vi "TRAJECTORY_CREATE_PATHFINDER_BEGIN.vi"() -> (0 "Path calculation error":errorcluster, 2 "Trajectory Items":i32, 3 "TotalTImeSecs":dbl)   [LabVIEW 2019]
uses:
  <vilib>/Rock Robotics/WPI/ThirdParty/JAS_Junk/JaciPathFinderLib/VIs/Waypoint.ctl
  <vilib>/Rock Robotics/WPI/ThirdParty/JAS_Junk/TrajLib/TRAJECTORY.ctl
  <vilib>/Rock Robotics/WPI/ThirdParty/JAS_Junk/TrajLib/TRAJ_STATE.ctl
  <vilib>/Rock Robotics/WPI/ThirdParty/JAS_Junk/TrajLib/POSE2D.ctl
  <vilib>/Rock Robotics/WPI/ThirdParty/JAS_Junk/TrajLib/TRANSLATION2D.ctl
  <vilib>/Rock Robotics/WPI/ThirdParty/JAS_Junk/TrajLib/ROTATION2D.ctl
  <vilib>/Rock Robotics/WPI/ThirdParty/JAS_Junk/TrajLib/Trajectory_Library.lvlib
  <vilib>/Rock Robotics/WPI/ThirdParty/JAS_Junk/JaciPathFinderLib/Pathfinder.lvlib
panel:
  out "TRAJECTORY":T1 {"TotalTImeSecs" format="%20.3f"}
  in  "Waypoints":T6[](array[typedef])=[{"x"=15.0, "y"=105.0, "angle"=-45.0}, {"x"=105.0, "y"=65.0, "angle"=0.0}, {"x"=210.0, "y"=106.0, "angle"=45.0}]
  in  "wheelbase_width":dbl=20.866
  in  "sample_count":i32=10000
  in  "Path Results\ndT":dbl=0.02 format="%7.3f"
  in  "max_jerk":dbl=50.0
  in  "max_acceleration":dbl=20.0
  in  "max_velocity":dbl=40.0
  # "TRAJECTORY CONFIGURATION"
  # "TRAJECTORY DEFINITION"
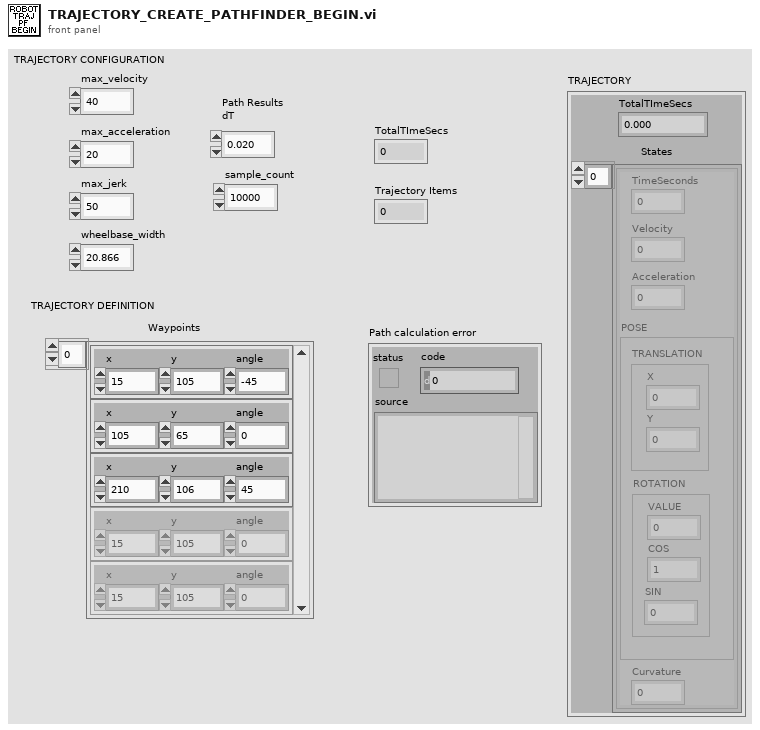
[diagram p1: front panel]
types:
  T1 = typedef "Trajectory_Library.lvlib/TRAJECTORY.ctl" = cluster{"TotalTImeSecs":dbl, "States":T2[]}
  T2 = typedef "Trajectory_Library.lvlib/TRAJ_STATE.ctl" = cluster{"TimeSeconds":dbl, "Velocity":dbl, "Acceleration":dbl, "POSE":T3, "Curvature":dbl}
  T3 = typedef "Trajectory_Library.lvlib/POSE2D.ctl" = cluster{"TRANSLATION":T4, "ROTATION":T5}
  T4 = typedef "Trajectory_Library.lvlib/TRANSLATION2D.ctl" = cluster{"X":dbl, "Y":dbl}
  T5 = typedef "Trajectory_Library.lvlib/ROTATION2D.ctl" = cluster{"VALUE":dbl, "COS":dbl, "SIN":dbl}
  T6 = typedef "Pathfinder.lvlib/Waypoint.ctl" = cluster{"x":dbl, "y":dbl, "angle":dbl}
  T7 = typedef "Pathfinder.lvlib/Segment.ctl" = cluster{"dt":dbl, "x":dbl, "y":dbl, "position":dbl, "velocity":dbl, "acceleration":dbl, "jerk":dbl, "heading":dbl}
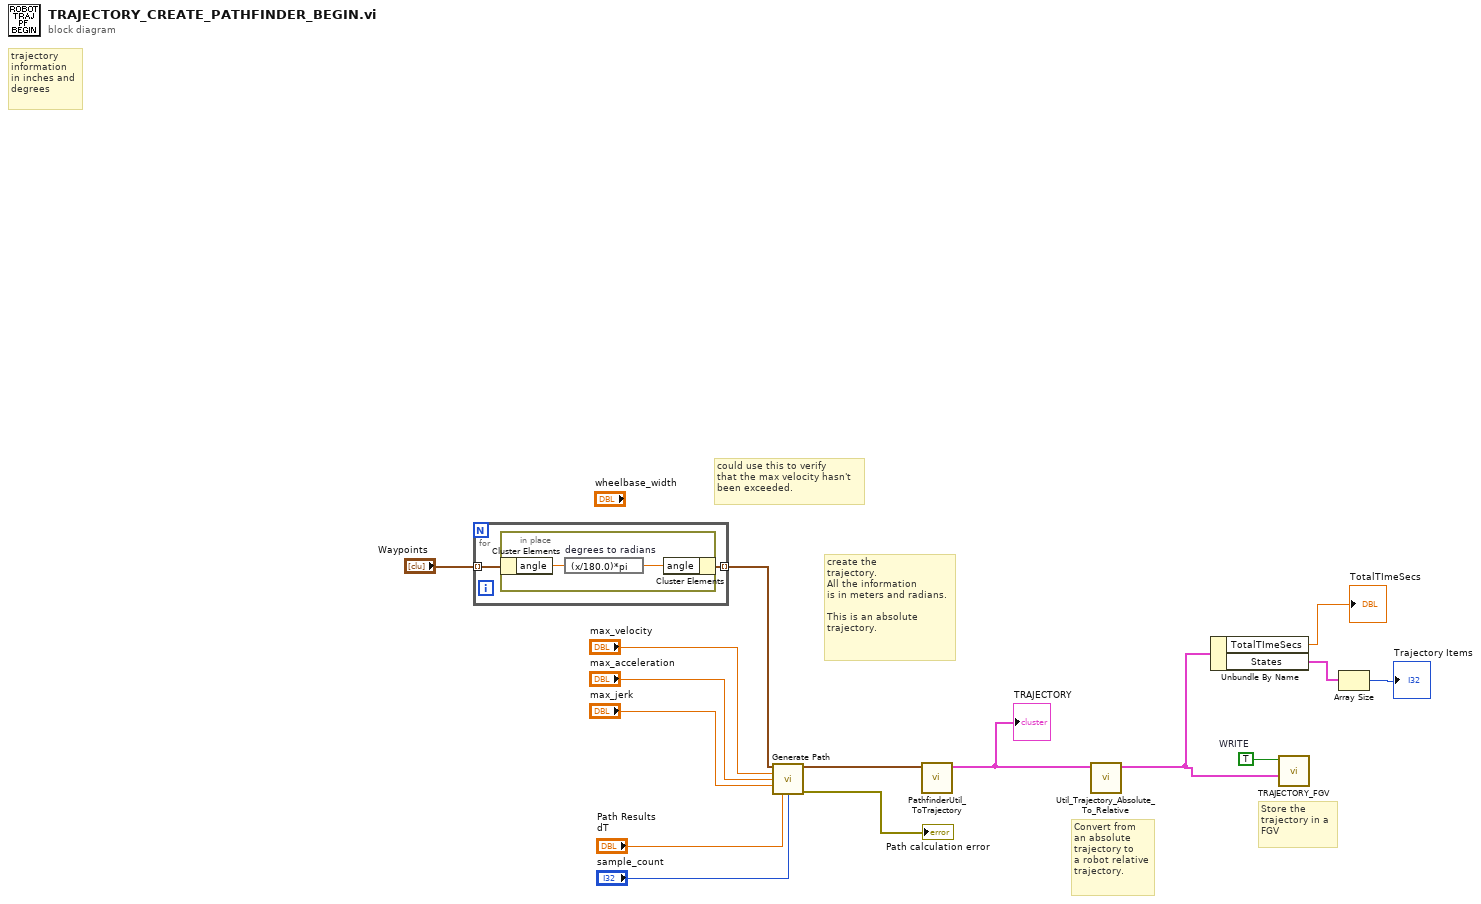
[diagram p0: block diagram]
diagram:
  w15 = TRUE  # WRITE
  # "could use this to verify\nthat the max velocity hasn't\nbeen exceeded."
  # "Store the\ntrajectory in a \nFGV"
  # "Convert from\nan absolute\ntrajectory to\na robot relative\ntrajectory."
  # "create the\ntrajectory.\nAll the information\nis in meters and radians.\n\nThis is an absolute \ntrajectory."
  # "trajectory\ninformation\nin inches and\ndegrees"
  n1 = for {
    tunnel: "Waypoints" -> [w17] mode=indexing
    tunnel: [w16] -> w9 mode=indexing
    n2 = in-place {
      n3 = in-place-cluster #1(w17) -> ("angle"=w19:dbl)
      n4 = expression code="(x/180.0)*pi" "degrees to radians"(w19) -> (w18:dbl)
      n5 = in-place-cluster #1("angle"=w18) -> (w16:T6)
    }
  }
  n6 = call <vilib>:"Generate Path.vi"("path"=w9, "max_velocity"="max_velocity", "max_acceleration"="max_acceleration", "max_jerk"="max_jerk", "dt (.001)"="Path Results\ndT", "sample_count (100000)"="sample_count") -> ("Segments"=w3:T7[], "error out"=→"Path calculation error":errorcluster)  [unwired: 8 in]
  n7 = call <vilib>:"PathfinderUtil_ToTrajectory.vi"("Pathfinder Path"=w3) -> ("TRAJECTORY"=w1:T1)  [unwired: 10 in]
  "TRAJECTORY" <- w1
  n8 = call <vilib>:"Util_Trajectory_Absolute_To_Relative.vi"("absTRAJECTORY"=w1) -> ("outputRelativeTRAJECTORY"=w11:T1)  [unwired: 10 in]
  n9 = Unbundle By Name(w11) -> ("TotalTImeSecs"=→"TotalTImeSecs":dbl, "States"=w13:T2[])
  n10 = call "TRAJECTORY_FGV.vi"("inTRAJECTORY"=w11, "WRITE"=w15) -> ()  [unwired: 9 in, 1 out]
  n11 = Array Size(array=w13) -> (size(s)=→"Trajectory Items":i32)
